vi "gyroConvert.vi"(8 "turnThis (-180 to 180)":dbl, 11 "angle (-180 to 180)":dbl) -> (0 "turnRight":bool, 3 "neededAngle (-180 to 180)":dbl)   [LabVIEW 2016]
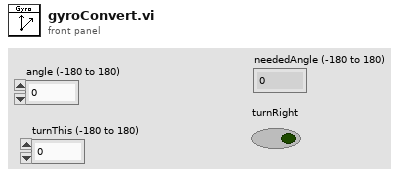
[diagram p1: front panel]
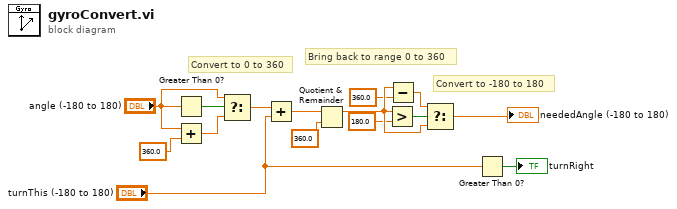
[diagram p0: block diagram]
diagram:
  # "Convert to -180 to 180"
  # "Bring back to range 0 to 360"
  # "Convert to 0 to 360"
  n1 = Greater Than 0?(x="angle (-180 to 180)") -> (x > 0?=w15:bool)
  n2 = Add(x="angle (-180 to 180)", y=360.0) -> (x+y=w14:dbl)
  n3 = Select(t="angle (-180 to 180)", s=w15, f=w14) -> (s? t:f=w11:dbl)
  n4 = Add(x=w11, y="turnThis (-180 to 180)") -> (x+y=w10:dbl)
  n5 = Quotient & Remainder(x=w10, y=360.0) -> (x-y*floor(x/y)=w8:dbl)  [unwired: 1 out]
  n6 = Greater?(x=w8, y=180.0) -> (0:w6:bool)
  n7 = Subtract(x=w8, y=360.0) -> (x-y=w5:dbl)
  n8 = Select(t=w5, s=w6, f=w8) -> (s? t:f=→"neededAngle (-180 to 180)":dbl)
  n9 = Greater Than 0?(x="turnThis (-180 to 180)") -> (x > 0?=→"turnRight":bool)
